vi "OuterLoopClock.vi"(10 "OuterLoopClockIRQ":refnum<class "IIRQ.lvclass">, 11 "UserEvents":refnum<class "UserEvents.lvclass">) -> ()   [LabVIEW 2016]
uses:
  UserEvents/UserEvents.lvclass
  Common_RT_FPGA/IIRQ/IIRQ.lvclass
  UserEvents/UserEvents.lvclass/UserEvents.ctl
  Commands/UpdateCommand/UpdateCommand.lvclass
  D:/Code/ts_M1M3Support/Commands/Command/Command.lvclass
  Types/ProcessCommandEvent.ctl
  Commands/Command/Command.lvclass
  Types/M1M3SupportTypes.lvlib
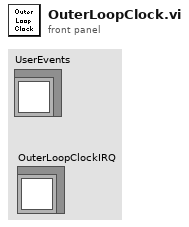
[diagram p1: front panel]
types:
  T1 = typedef "M1M3SupportTypes.lvlib/ProcessCommandEvent.ctl" = cluster{"Command":refnum<class "Command.lvclass">}
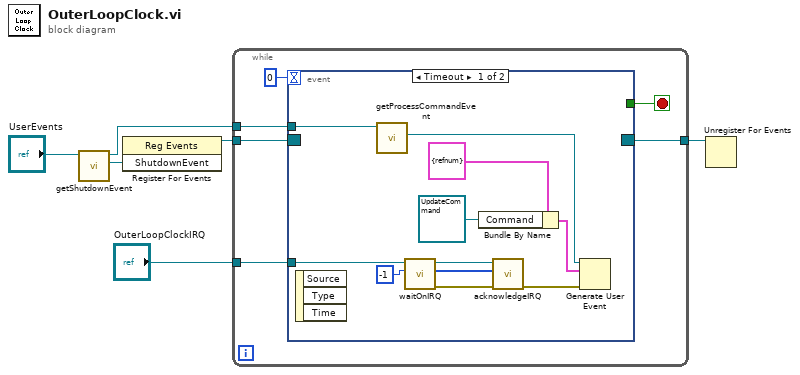
[diagram p0: block diagram]
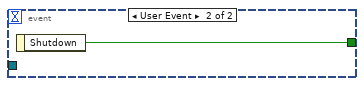
[diagram p2: hidden frame]
diagram:
  n1 = call "getShutdownEvent.vi"("UserEvents in"="UserEvents") -> ("ShutdownEvent"=w6:refnum<user-event>, "UserEvents out"=w4:refnum<class "UserEvents.lvclass">)  [unwired: 9 in]
  n2 = register-events(w6) -> (reference out=w5:refnum<event-registration>)  [unwired: 2 in, 1 out]
  n3 = while {
    tunnel: w5 -> [w11]
    tunnel: [w10] -> w3
    tunnel: w4 -> [w8]
    tunnel: "OuterLoopClockIRQ" -> [w7]
    stop <- w9 stop-if-true
    n4 = event shown="[0] Timeout" {
      selector: w11 -> [_ _]
      dyn-events: [_ _] -> w10
      timeout: 0 -> [_ _]
      tunnel: [_ w24] -> w9
      tunnel: w8 -> [w23 _]
      tunnel: w7 -> [w17 _]
      event Timeout {
        n5 = event-data() -> ()  [unwired: 1 in, 3 out]
        n6 = call "getProcessCommandEvent.vi"("UserEvents in"=w23) -> ("ProcessCommandEvent"=w19:refnum<user-event>)  [unwired: 9 in, 1 out]
        n7 = call-dynamic "waitOnIRQ.vi"("Timeout"=-1 ("Timeout (ms)"), "IIRQ in"=w17) -> ("error out"=w14:errorcluster, "IRQs"=w16:i32[], "IIRQ out"=w15:refnum<class "IIRQ.lvclass">)  [unwired: 6 in, 1 out]
        n8 = Bundle By Name(cluster=T1 {"Command"=refnum} ("ProcessCommandEvent"), "Command"=refnum<class "UpdateCommand.lvclass"> refnum ("UpdateCommand.lvclass")) -> (w20:T1)
        n9 = call-dynamic "acknowledgeIRQ.vi"("error in (no error)"=w14, "IRQs"=w16, "IIRQ in"=w15) -> ("error out"=w13:errorcluster)  [unwired: 7 in, 1 out]
        n10 = Generate User Event(user event=w19, event data cluster=w20, error in=w13) -> ()  [unwired: 1 in, 2 out]
      }
      event User Event {
        n11 = event-data() -> ("Shutdown"=w24:bool)  [unwired: 1 in]
      }
    }
  }
  n12 = Unregister For Events(event registration refnum=w3) -> ()  [unwired: 1 in, 1 out]
